vi "runDone.vi"(9 "desiredTime":i32, 11 "startTimer":bool) -> (3 "doneRunning?":bool)   [LabVIEW 2017]
uses:
  <vilib>/FRCT Team# 3937  Breakaway/Memory Library/memLib.lvlib
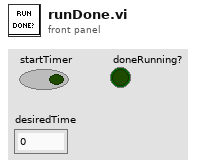
[diagram p1: front panel]
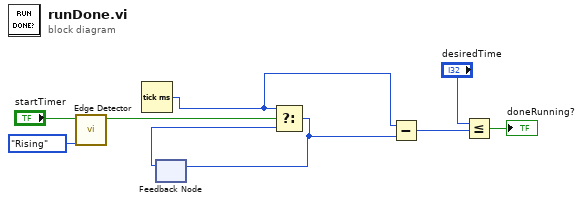
[diagram p0: block diagram]
diagram:
  n1 = call <vilib>:"Edge Detector.vi"("Mode"=enum16{"Rising", "Falling", "Any"}."Rising", "Input"="startTimer") -> ("Output"=w2:bool)  [unwired: 9 in]
  n2 = Tick Count (ms)() -> (millisecond timer value=w8:u32)
  n3 = feedback #1() -> (w9:u32)  [unwired: 1 in]
  n4 = Select(t=w8, s=w2, f=w9) -> (s? t:f=w7:u32)
  n5 = feedback-in #1(w7) -> ()
  n6 = Subtract(x=w8, y=w7) -> (x-y=w5:u32)
  n7 = Less Or Equal?(x="desiredTime", y=w5) -> (x <= y?=→"doneRunning?":bool)
